vi "Data Deserialize (Data).vi"(8 "error in (no error)":errorcluster, 10 "Data":refnum<data-value>, 11 "Data DVR in":refnum<data-value>) -> (0 "error out":errorcluster, 2 "Data out":refnum<data-value>, 3 "Data DVR out":refnum<data-value>)   [LabVIEW 2012, in "MDSplus.lvlib"]
uses:
  <vilib>/MDSplus/Library/MDSplus.lvlib
  <vilib>/MDSplus/Classes/Data_Class/Data.lvclass
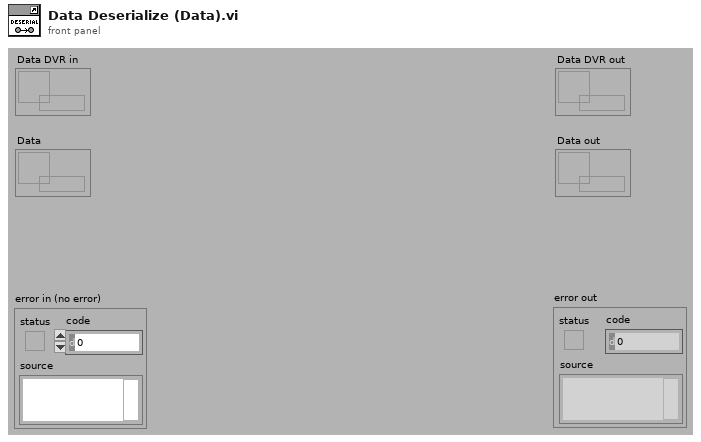
[diagram p1: front panel]
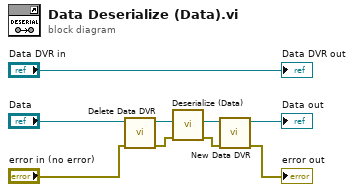
[diagram p0: block diagram]
diagram:
  n1 = call <vilib>:"Delete Data DVR.vi"("error in (no error)"="error in (no error)", "Data DVR in"="Data") -> ("error out"=w4:errorcluster, "Data out"=w3:refnum<class "Data.lvclass">)  [unwired: 8 in]
  n2 = call <vilib>:"Deserialize (Data).vi"("error in (no error)"=w4, "Data"=w3) -> ("error out"=w9:errorcluster, "Returned data out"=w2:refnum<class "Data.lvclass">)  [unwired: 7 in, 1 out]
  n3 = call <vilib>:"New Data DVR.vi"("error in (no error)"=w9, "Data in"=w2) -> ("error out"=→"error out":errorcluster, "Data DVR out"=→"Data out":refnum<data-value>)  [unwired: 8 in]
  "Data DVR out" <- "Data DVR in"
